vi "DSF.Engine.Framework.Create.Cache.vi"(8 "error in (no error)":errorcluster, 11 "Framework in":refnum<class "DSF.Engine.Framework.lvclass">) -> (0 "error out":errorcluster, 3 "Framework out":refnum<class "DSF.Engine.Framework.lvclass">)   [LabVIEW 2017, in "DSF.Engine.lvlib" / "DSF.Engine.Framework.lvclass"]
uses:
  DSF.Engine.Framework.lvclass
  Transfer/DSF.Engine.Transfer Group.lvclass
  Transfer/DSF.Engine.Transfer.lvclass
  DSF.Engine.Framework.lvclass/DSF.Engine.Framework.ctl
  Cache/DSF.Engine.Memory.Cache.lvclass
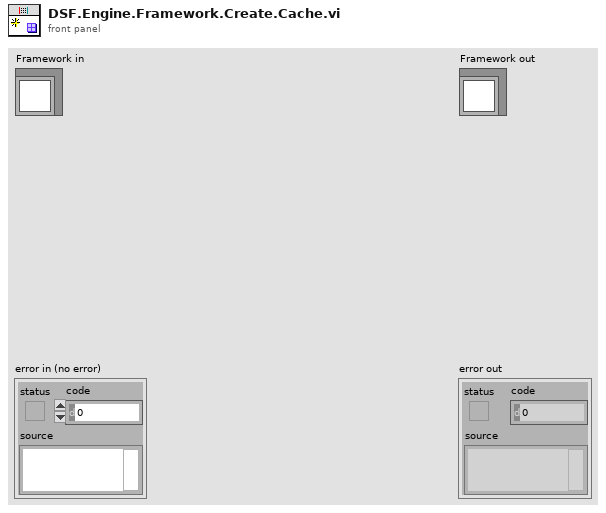
[diagram p1: front panel]
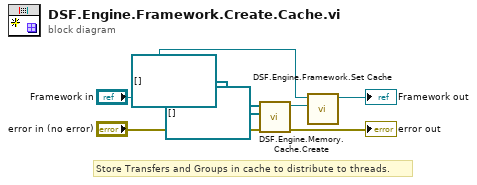
[diagram p0: block diagram]
diagram:
  # "Store Transfers and Groups in cache to distribute to threads."
  n1 = call "DSF.Engine.Memory.Cache.Create.vi"("error in (no error)"="error in (no error)", "Transfers"=refnum<class "DSF.Engine.Transfer.lvclass">[] [], "Transfers Groups"=refnum<class "DSF.Engine.Transfer Group.lvclass">[] []) -> ("error out"=→"error out":errorcluster, "Cache out"=w7:refnum<class "DSF.Engine.Memory.Cache.lvclass">)  [unwired: 7 in]
  n2 = call "DSF.Engine.Framework.Set Cache.vi"("Cache"=w7, "Framework in"="Framework in") -> ("Framework out"=→"Framework out":refnum<class "DSF.Engine.Framework.lvclass">)  [unwired: 9 in]
